vi "ADSR.vi"(4 "Gate":bool, 6 "Trigger":bool, 8 "S/R":fxp<+,16,0>=1.52587890625e-05, 9 "Sustain":fxp<+,16,0>=0.6999969482421875, 10 "1/Decay":fxp<+,16,0>=1.52587890625e-05, 11 "1/Attack":fxp<+,16,0>=1.52587890625e-05) -> (5 "Amount?":bool, 7 "Sample Out":fxp<+,8,0>)   [LabVIEW 2015]
doc: "Like the traditional ADSR, this VI outputs a simple Attack-Decay-Sustain-Release envelope every time 'Trigger' is toggled, until 'Gate' turns off."
uses:
  TypeDefs FPGA/EG Shape Enum.ctl
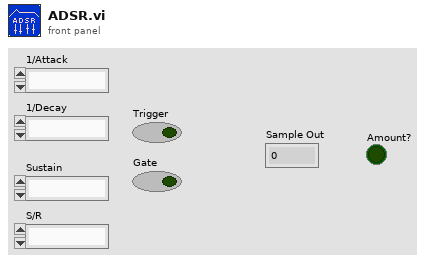
[diagram p1: front panel]
types:
  T1 = typedef "EG Shape Enum.ctl" = enum16{"Idle", "Attack", "Decay", "Sustain", "Release"}
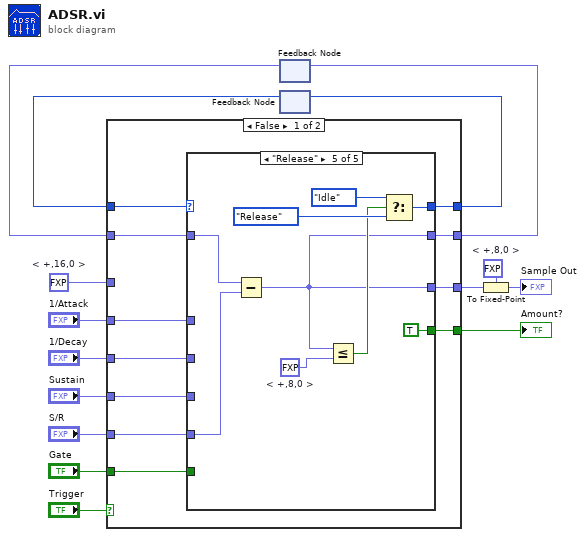
[diagram p0: block diagram]
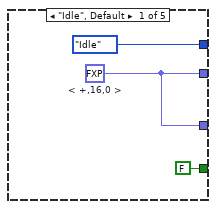
[diagram p2: hidden frame]
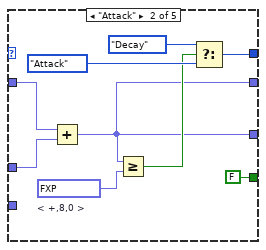
[diagram p3: hidden frame]
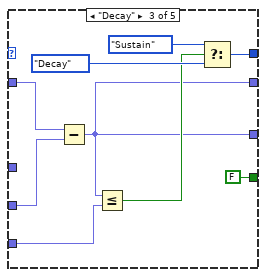
[diagram p4: hidden frame]
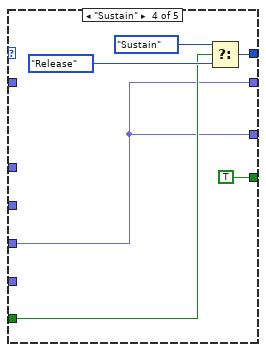
[diagram p5: hidden frame]
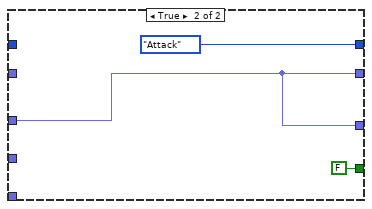
[diagram p6: hidden frame]
diagram:
  w6 = fxp<+,8,0> 0.0  # < +,8,0 >
  w9 = fxp<+,16,0> 0.0  # < +,16,0 >
  n1 = feedback #1() -> (w2:fxp<+,16,0>)  [unwired: 1 in]
  n2 = feedback #2() -> (w4:T1)  [unwired: 1 in]
  n3 = case shown="False" "Trigger" {
    tunnel: w9 -> [_ w64]
    tunnel: [w22 EG_Shape_Enum."Attack" ("EG States")] -> w5
    tunnel: w4 -> [w26 _]
    tunnel: "1/Attack" -> [w25 _]
    tunnel: "1/Decay" -> [w24 _]
    tunnel: "Sustain" -> [w18 _]
    tunnel: "S/R" -> [w23 _]
    tunnel: [w21 w64] -> w3
    tunnel: w2 -> [w17 _]
    tunnel: [w20 w64] -> w8
    tunnel: "Gate" -> [w19 _]
    tunnel: [w16 FALSE] -> w1
    frame False {
      n4 = case shown="\"Release\"" w26 {
        tunnel: w17 -> [_ w34 w43 _ w57]
        tunnel: w25 -> [_ w32 _ _ _]
        tunnel: w24 -> [_ _ w41 _ _]
        tunnel: w18 -> [_ _ w42 w49 _]
        tunnel: w23 -> [_ _ _ _ w56]
        tunnel: [EG_Shape_Enum."Idle" ("EG States") w36 w44 w51 w59] -> w22
        tunnel: [w28 w31 w40 w49 w55] -> w21
        tunnel: [w28 w31 w40 w49 w55] -> w20
        tunnel: w19 -> [_ _ _ w50 _]
        tunnel: [FALSE FALSE FALSE TRUE TRUE] -> w16
        frame "Idle", Default {
          w28 = fxp<+,16,0> 0.0  # < +,16,0 >
        }
        frame "Attack" {
          w33 = fxp<+,8,0> 0.99609375  # < +,8,0 >
          n5 = Add(x=w34, y=w32) -> (x+y=w31:fxp<+,16,0>)
          n6 = Greater Or Equal?(x=w31, y=w33) -> (x >= y?=w35:bool)
          n7 = Select(t=EG_Shape_Enum."Decay" ("EG States"), s=w35, f=EG_Shape_Enum."Attack" ("EG States")) -> (s? t:f=w36:T1)
        }
        frame "Decay" {
          n8 = Subtract(x=w43, y=w41) -> (x-y=w40:fxp<+,16,0>)
          n9 = Less Or Equal?(x=w40, y=w42) -> (x <= y?=w45:bool)
          n10 = Select(t=EG_Shape_Enum."Sustain" ("EG States"), s=w45, f=EG_Shape_Enum."Decay" ("EG States")) -> (s? t:f=w44:T1)
        }
        frame "Sustain" {
          n11 = Select(t=EG_Shape_Enum."Sustain" ("EG States"), s=w50, f=EG_Shape_Enum."Release" ("EG States")) -> (s? t:f=w51:T1)
        }
        frame "Release" {
          w58 = fxp<+,8,0> 0.0  # < +,8,0 >
          n12 = Subtract(x=w57, y=w56) -> (x-y=w55:fxp<+,16,0>)
          n13 = Less Or Equal?(x=w55, y=w58) -> (x <= y?=w60:bool)
          n14 = Select(t=EG_Shape_Enum."Idle" ("EG States"), s=w60, f=EG_Shape_Enum."Release" ("EG States")) -> (s? t:f=w59:T1)
        }
      }
    }
    frame True {
    }
  }
  "Amount?" <- w1
  n15 = feedback-in #1(w3) -> ()
  n16 = feedback-in #2(w5) -> ()
  n17 = To Fixed-Point(fixed-point type=w6, number=w8) -> (fixed-point=→"Sample Out":fxp<+,8,0>)
